vi "converting to mp4.vi"(8 "error in (no error)":errorcluster) -> (0 "error out":errorcluster, 2 "media source":string, 3 "script string":string)   [LabVIEW 2012]
uses:
  Controls-Webcam/VLC Var.ctl
panel:
  in  "VLC Variables In":T1
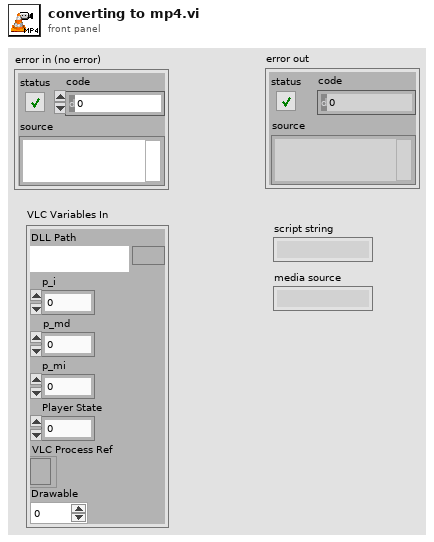
[diagram p1: front panel]
types:
  T1 = typedef "VLC Var.ctl" = cluster{"DLL Path":path, "p_i":i32, "p_md":i32, "p_mi":i32, "Player State":i32, "VLC Process Ref":refnum<k24>, "Drawable":i32}
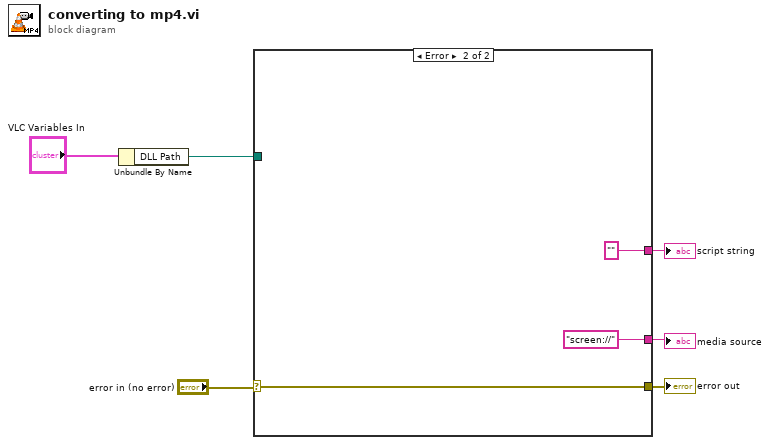
[diagram p0: block diagram]
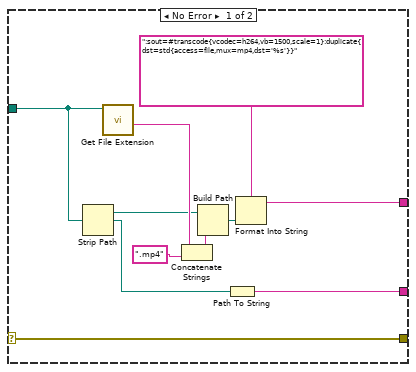
[diagram p2: hidden frame]
diagram:
  n1 = Unbundle By Name("VLC Variables In") -> ("DLL Path"=w2:path)
  n2 = case shown="Error" "error in (no error)" {
    selector: "error in (no error)" -> [w7 w17]
    tunnel: [w16 ""] -> w6
    tunnel: [w15 "screen://"] -> w5
    tunnel: w2 -> [w8 _]
    tunnel: [w7 w17] -> w3
    frame No Error {
      n3 = Strip Path(path=w8) -> (stripped path=w10:path)  [unwired: 1 out]
      n4 = call <vilib>:"Get File Extension.vi"("file"=w8) -> ("filename without extension"=w12:string)  [unwired: 7 in, 3 out]
      n5 = Concatenate Strings(w12, ".mp4" ("string")) -> (w13:string)
      n6 = Build Path(base path=w10, name or relative path=w13) -> (appended path=w11:path)
      n7 = Path To String(path=w8) -> (string=w15:string)
      n8 = Format Into String(format string=":sout=#transcode{vcodec=h264,vb=1500,scale=1}:duplicate{dst=std{access=file,mux=mp4,dst='%s'}}", w11) -> (resulting string=w16:string)  [unwired: 2 in, 1 out]
    }
    frame Error {
    }
  }
  "media source" <- w5
  "script string" <- w6
  "error out" <- w3
